vi "camera_release configuration_stop.vi"(2 "Image Memory":T1, 3 "Detektionskamera":T2) -> (0 "error out":errorcluster, 1 "status":bool)   [LabVIEW 2009]
uses:
  <vilib>/userDefined/High Color/IMAQdx.ctl
  <vilib>/vision/Image Controls.llb/IMAQ Image.ctl
  <vilib>/vision/driver/NI_Vision_Acquisition_Software.lvlib
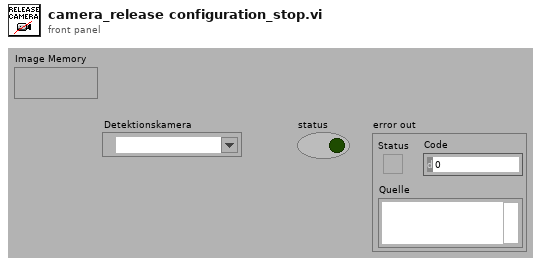
[diagram p1: front panel]
types:
  T1 = typedef "IMAQ Image.ctl" = refnum<image>
  T2 = typedef "IMAQdx.ctl" = refnum<k21>
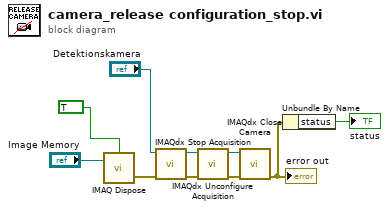
[diagram p0: block diagram]
diagram:
  n1 = call "IMAQ Dispose"("All Images? (No)"=TRUE, "Image"="Image Memory") -> ("error out"=w9:errorcluster)  [unwired: 4 in]
  n2 = call <vilib>:"IMAQdx Stop Acquisition.vi"("error in"=w9, "Session In"="Detektionskamera") -> ("error out"=w5:errorcluster, "Session Out"=w4:T2)  [unwired: 8 out]
  n3 = call <vilib>:"IMAQdx Unconfigure Acquisition.vi"("error in"=w5, "Session In"=w4) -> ("error out"=w2:errorcluster, "Session Out"=w3:T2)  [unwired: 8 out]
  n4 = call <vilib>:"IMAQdx Close Camera.vi"("error in"=w2, "Session In"=w3) -> ("error out"=w7:errorcluster)  [unwired: 9 out]
  "error out" <- w7
  n5 = Unbundle By Name(w7) -> ("status"=→"status":bool)
